vi "Serial Read FOR Arduino.vi"() -> ()   [LabVIEW 2024]
doc: "This example performs writes and reads on a serial port, as directed by the user. You can press the Write and Read buttons, and change the Read Count, while the example is running.\n\nThe parameters set for the serial port must match the parameters of the connected instrument or device. In this example, the Read Count parameter specifies the number of bytes that the serial port reads. If there were more bytes at the port than the specified number, those bytes would not be read. If there were less bytes at the port than the specified number, you would receive a timeout error.\n\nThis example expands upon the flow control options for XON and XOFF, allowing the user to choose those control characters. Also, the user can enable or disable a termination character. Some devices require a termination character in order to identify the end of command strings. Some devices send a termination character to signify the end of data to be read. This example shows how you can end the Read operation once a termination character is detected in the buffer and/or append a termination character at the end of the Write data."
uses:
  support/Serial - Settings.ctl
  <vilib>/Instr/_visa.llb/VISA Configure Serial Port (Instr).vi
panel:
  out "size(s)":i32[](array[numeric])
  out "element 3":dbl
  out "element 2":dbl
  out "element":dbl
  out "Waveform Graph":dbl[][](graph)
  in  "Read Count 2":u32=1000
  out "Numeric":i32
  in  "Termination Character":u8=10 format="%.0x"
  in  "End Write on Termination Character?":bool=TRUE
  in  "Stop":bool
  in  "Command":string="*IDN?"
  in  "Write":bool
  in  "Serial Settings":T1={"baud rate"=115200, "data bits"=8, "parity"=enum."None", "stop bits"=10, "flow control"=0} {"flow control" items=["None"=0, "XON/XOFF"=1, "RTS/CTS"=2, "DTR/DSR"=4]; "stop bits" items=["1.0"=10, "1.5"=15, "2.0"=20]; "data bits" min=5 max=8 step=1; "baud rate" items=["75"=75, "110"=110, "134"=134, "150"=150, "300"=300, "600"=600, "1200"=1200, "1800"=1800, "2400"=2400, "4800"=4800, "7200"=7200, "9600"=9600, "14400"=14400, "19200"=19200, "28800"=28800, "38400"=38400, "56000"=56000, "57600"=57600, "115200"=115200, "128000"=128000, "230400"=230400]}
  in  "End Read on Termination Character?":bool=TRUE
  in  "VISA resource name":refnum<visa-resource-name>="COM1"
  # "Overview: Demonstrates the use of the VISA functions to write commands to and read responses from a serial instrument continuously in a loop.\nRequirements: NI-VISA Driver\nInstructions:\n1. Run the VI.\n2. Specify a Command and click the Write button.\n3. Read a Response by clicking the Read button.\n4. Click Stop to stop the VI."
  # "0xA is equivalent to a '\\n' character, which is a line feed."
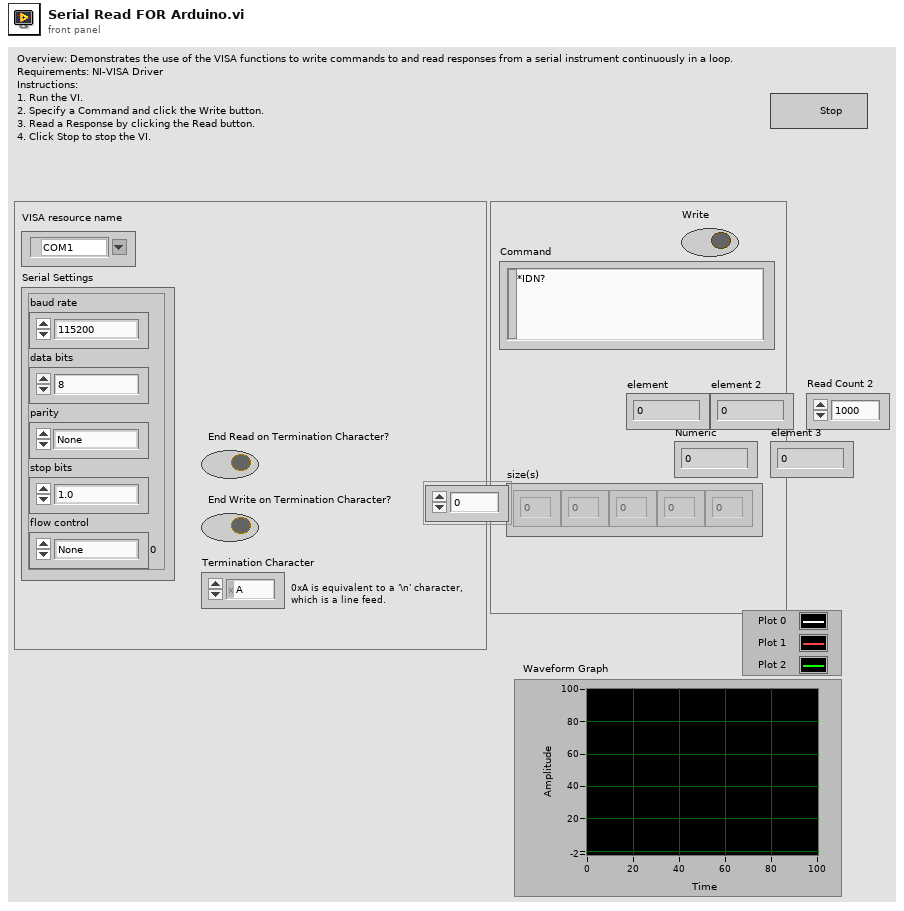
[diagram p1: front panel]
types:
  T1 = typedef "Serial - Settings.ctl" = cluster{"baud rate":u32, "data bits":u16, "parity":enum16{"None", "Odd", "Even", "Mark", "Space"}, "stop bits":u16, "flow control":u16}
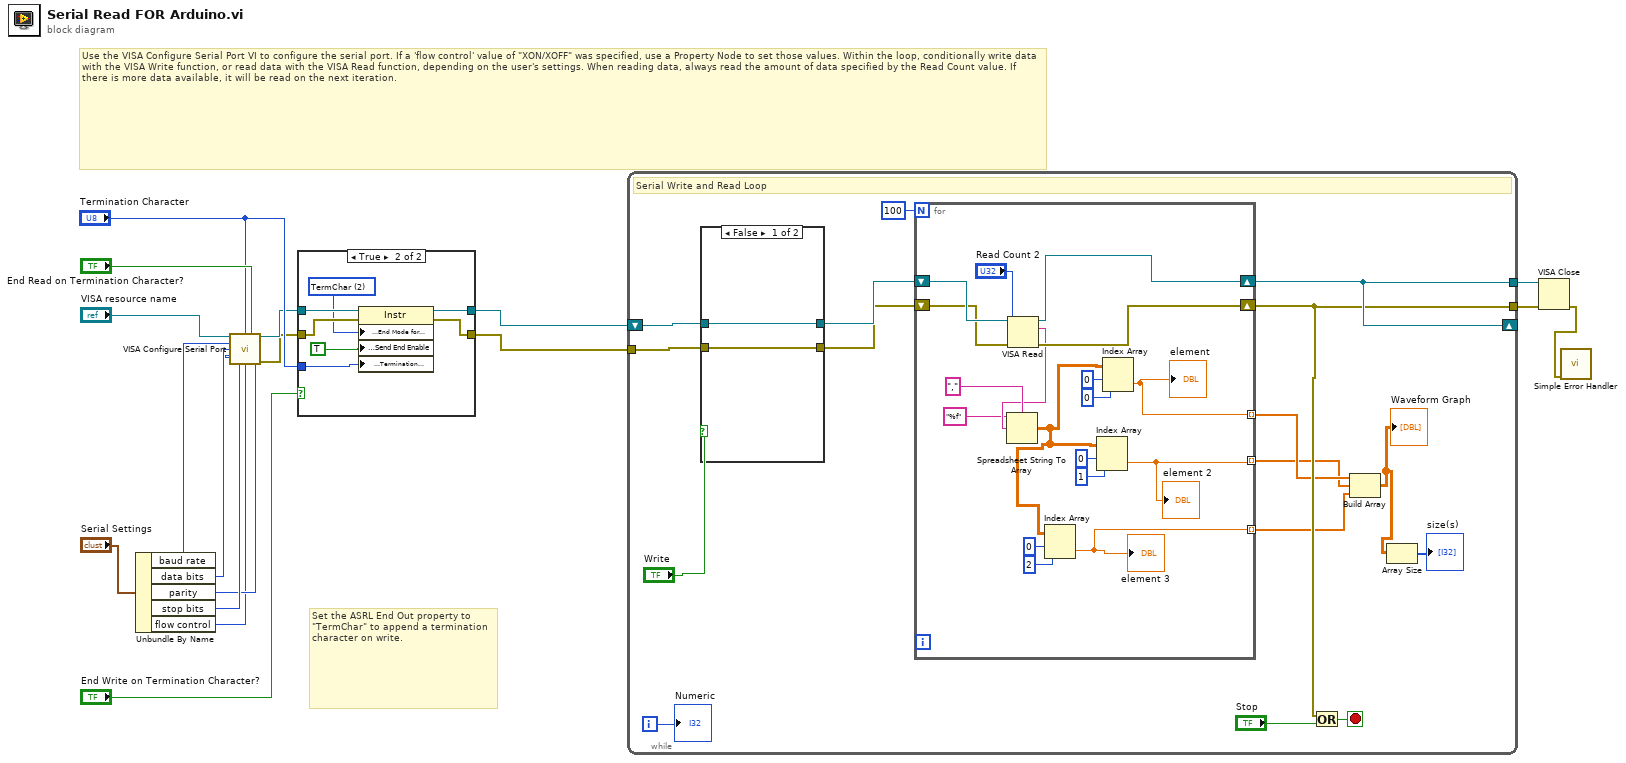
[diagram p0: block diagram]
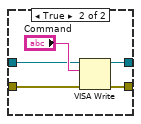
[diagram p3: hidden frame]
diagram:
  # "Set the ASRL End Out property to \"TermChar\" to append a termination character on write."
  # "Use the VISA Configure Serial Port VI to configure the serial port. If a 'flow control' value of \"XON/XOFF\" was specified, use a Property Node to set those values. Within the loop, conditionally write data with the VISA Write function, or read data with the VISA Read function, depending on the user's settings. When reading data, always read the amount of data specified by the Read Count value. If there is more data available, it will be read on the next iteration."
  n1 = Unbundle By Name("Serial Settings") -> ("baud rate"=w13:u32, "data bits"=w14:u16, "parity"=w15:enum16{"None", "Odd", "Even", "Mark", "Space"}, "stop bits"=w16:u16, "flow control"=w10:u16)
  n2 = call-poly "VISA Configure Serial Port"("VISA resource name"="VISA resource name", "termination char\n(0xA = '\\n' = LF)"="Termination Character", "Enable Termination\nChar (T)"="End Read on Termination Character?", "baud rate (9600)"=w13, "data bits (8)"=w14, "parity (0:none)"=w15, "stop bits (10: 1 bit)"=w16, "flow control (0:none)"=w10) -> ("VISA resource name out"=w5:refnum<visa-resource-name>, "error out"=w4:errorcluster)  [unwired: 2 in, 4 out]
  n3 = case shown="True" "End Write on Termination Character?" {
    tunnel: w5 -> [w18 w26]
    tunnel: w4 -> [w19 w25]
    tunnel: [w18 w24] -> w8
    tunnel: [w19 w23] -> w9
    tunnel: "Termination Character" -> [_ w21]
    frame False {
    }
    frame True {
      w22 = u16 2 items=["None", "LastBit", "TermChar", "Break"] ("Serial Settings:Serial End Mode for Writes")
      n4 = property class="Instr"(reference=w26, error in=w25, "Serial Settings:End Mode for Writes"=w22, "Message Based Settings:Send End Enable"=TRUE, "Message Based Settings:Termination Character"=w21) -> (reference out=w24:refnum<visa-resource-name>, error out=w23:errorcluster)
    }
  }
  n5 = while {
    shift-right: [w34] -> _
    shift-left: w8 -> [w42]
    tunnel: w9 -> [w41]
    tunnel: [w33] -> w3
    tunnel: [w34] -> w2
    i -> [w37]
    stop <- w40 stop-if-true
    # "Serial Write and Read Loop"
    n6 = case shown="False" "Write" {
      tunnel: w42 -> [w62 w66]
      tunnel: w41 -> [w61 w65]
      tunnel: [w62 w64] -> w36
      tunnel: [w61 w63] -> w35
      frame False {
      }
      frame True {
        n7 = VISA Write(VISA resource name=w66, write buffer="Command", error in (no error)=w65) -> (VISA resource name out=w64:refnum<visa-resource-name>, error out=w63:errorcluster)  [unwired: 1 out]
      }
    }
    n8 = for {
      N: 100 -> [_]
      shift-right: [w56] -> w34
      shift-left: w36 -> [w59]
      shift-right: [w57] -> w33
      shift-left: w35 -> [w58]
      tunnel: [w48] -> w31 mode=indexing
      tunnel: [w47] -> w32 mode=indexing
      tunnel: [w43] -> w29 mode=indexing
      n9 = VISA Read(VISA resource name=w59, byte count="Read Count 2", error in (no error)=w58) -> (VISA resource name out=w56:refnum<visa-resource-name>, read buffer=w50:string, error out=w57:errorcluster)  [unwired: 1 out]
      n10 = Spreadsheet String To Array(delimiter (Tab)=",", format string="%f", spreadsheet string=w50) -> (array=w44:dbl[][])  [unwired: 1 in]
      n11 = Index Array(array=w44, index (row)=0, index (col)=2 ("disabled index (col)")) -> (element=w43:dbl)
      "element 3" <- w43
      n12 = Index Array(array=w44, index (row)=0, index (col)=1 ("disabled index (col)")) -> (element=w48:dbl)
      "element 2" <- w48
      n13 = Index Array(array=w44, index (row)=0, index (col)=0 ("disabled index (col)")) -> (element=w47:dbl)
      "element" <- w47
    }
    n14 = Or(x=w33, y="Stop") -> (x .or. y?=w40:bool)
    n15 = Build Array(w32, w31, w29) -> (w28:dbl[][])
    "Waveform Graph" <- w28
    n16 = Array Size(array=w28) -> (size(s)=→"size(s)":i32[])
    "Numeric" <- w37
  }
  n17 = VISA Close(VISA resource name=w2, error in (no error)=w3) -> (error out=w1:errorcluster)
  n18 = call <vilib>:"Simple Error Handler.vi"("error in (no error)"=w1) -> ()  [unwired: 1 in, 8 out]
